vi "Build sampling info (subVI).vi"(8 "error in (no error)":errorcluster, 10 "resolution (# of lines)":u32=800, 11 "baseband span":dbl=10000.0) -> (0 "error out":errorcluster, 1 "sampling info":cluster{"Fs":dbl, "#s":dbl}, 2 "FFT info":T1)   [LabVIEW 2023]
doc: "Converts the span and resolution to actual sampling frequency and # of samples to acquire. This VI also returns useful information about the acquisition time."
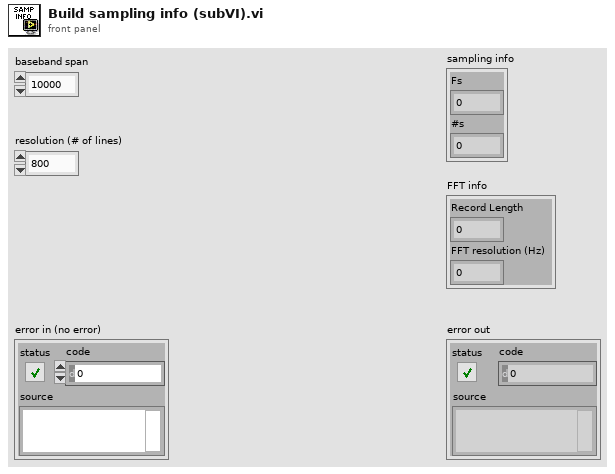
[diagram p1: front panel]
types:
  T1 = cluster{"Record Length":dbl, "FFT resolution (Hz)":dbl}
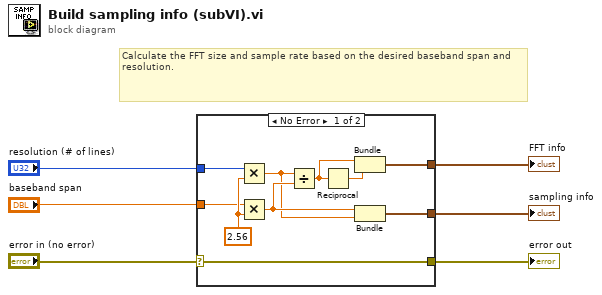
[diagram p0: block diagram]
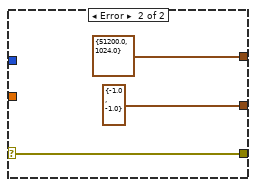
[diagram p2: hidden frame]
diagram:
  # "Calculate the FFT size and sample rate based on the desired baseband span and resolution."
  n1 = case shown="No Error" "error in (no error)" {
    selector: "error in (no error)" -> [w7 w19]
    tunnel: "resolution (# of lines)" -> [w11 _]
    tunnel: "baseband span" -> [w10 _]
    tunnel: [w7 w19] -> w3
    tunnel: [w9 cluster{dbl, dbl} {-1.0, -1.0}] -> w2
    tunnel: [w8 cluster{dbl, dbl} {51200.0, 1024.0}] -> w1
    frame No Error {
      w13 = 2.56 ("y")
      n2 = Multiply(x=w11, y=w13) -> (x*y=w12:dbl)
      n3 = Multiply(x=w10, y=w13) -> (x*y=w14:dbl)
      n4 = Divide(x=w12, y=w14) -> (x/y=w16:dbl)
      n5 = Reciprocal(x=w16) -> (1/x=w15:dbl)
      n6 = Bundle(w16, w15) -> (w8:cluster{dbl, dbl})  [unwired: 1 in]
      n7 = Bundle(w14, w12) -> (w9:cluster{dbl, dbl})  [unwired: 1 in]
    }
    frame Error {
    }
  }
  "error out" <- w3
  "FFT info" <- w1
  "sampling info" <- w2
